vi "Auton #3 one green bin begin.vi"   [LabVIEW 2014]
uses:
  Robot Global Data.vi
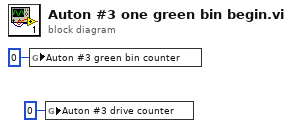
[diagram p0: block diagram]
diagram:
  n1 = global write "Robot Global Data.vi" "Auton #3 green bin counter"(i8 0 ("Auton #3 green bin counter")) -> ()
  n2 = global write "Robot Global Data.vi" "Auton #3 drive counter"(i16 0 ("Auton #3 drive counter")) -> ()
